vi "Set Channel.vi"(8 "error in (no error)":errorcluster, 10 "ADC Channel Selection":T1, 11 "LINX-ADS1256 in":refnum<class "LINX-ADS1256.lvclass">) -> (0 "error out":errorcluster, 3 "LINX-ADS1256 out":refnum<class "LINX-ADS1256.lvclass">)   [LabVIEW 2020, in "LINX-ADS1256.lvclass"]
uses:
  LINX-ADS1256.lvclass
  Channel Selection.ctl
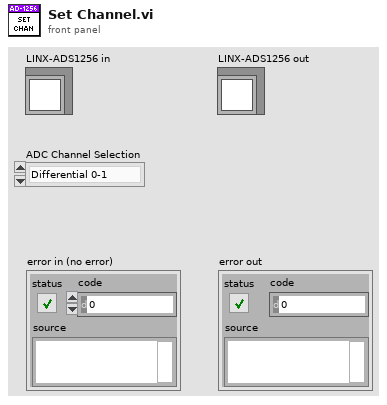
[diagram p1: front panel]
types:
  T1 = typedef "LINX-ADS1256.lvclass/Channel Selection.ctl" = enum16{"Differential 0-1", "Differential 2-3", "Differential 4-5", "Differential 6-7", "Single Ended 0", "Single Ended 1", "Single Ended 2", "Single Ended 3", "Single Ended 4", "Single Ended 5", "Single Ended 6", "Single Ended 7"}
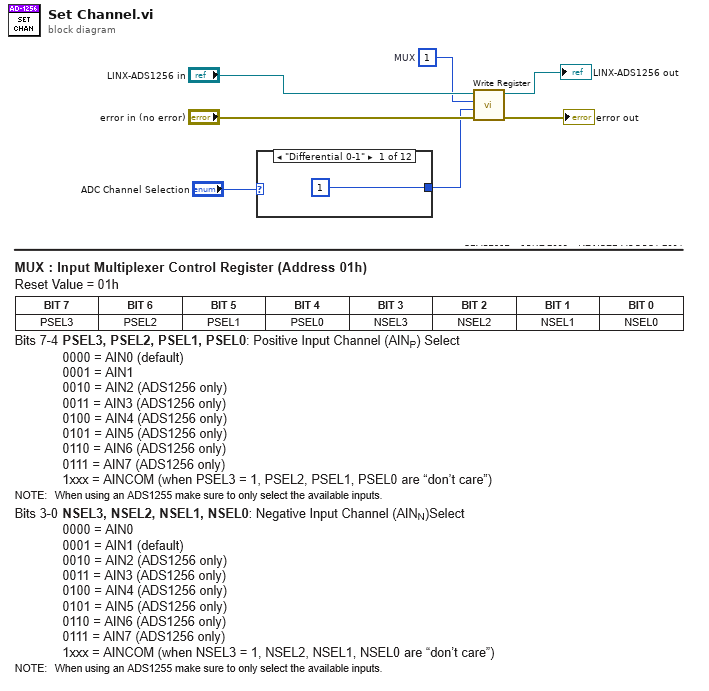
[diagram p0: block diagram]
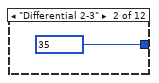
[diagram p2: hidden frame]
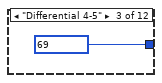
[diagram p3: hidden frame]
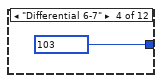
[diagram p4: hidden frame]
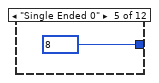
[diagram p5: hidden frame]
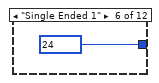
[diagram p6: hidden frame]
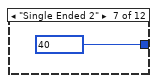
[diagram p7: hidden frame]
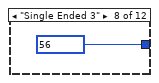
[diagram p8: hidden frame]
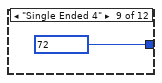
[diagram p9: hidden frame]
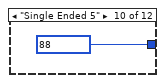
[diagram p10: hidden frame]
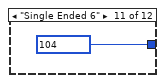
[diagram p11: hidden frame]
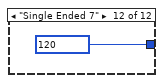
[diagram p12: hidden frame]
diagram:
  w4 = u8 1  # MUX
  n1 = case shown="\"Differential 0-1\"" "ADC Channel Selection" {
    tunnel: [u8 1 ("Data") u8 35 ("Data") u8 69 ("Data") u8 103 ("Data") u8 8 ("Data") u8 24 ("Data") u8 40 ("Data") u8 56 ("Data") u8 72 ("Data") u8 88 ("Data") u8 104 ("Data") u8 120 ("Data")] -> w1
    frame "Differential 0-1" {
    }
    frame "Differential 2-3" {
    }
    frame "Differential 4-5" {
    }
    frame "Differential 6-7" {
    }
    frame "Single Ended 0" {
    }
    frame "Single Ended 1" {
    }
    frame "Single Ended 2" {
    }
    frame "Single Ended 3" {
    }
    frame "Single Ended 4" {
    }
    frame "Single Ended 5" {
    }
    frame "Single Ended 6" {
    }
    frame "Single Ended 7" {
    }
  }
  n2 = call "Write Register.vi"("error in (no error)"="error in (no error)", "Data"=w1, "Register Address"=w4, "LINX-ADS1256 in"="LINX-ADS1256 in") -> ("error out"=→"error out":errorcluster, "LINX-ADS1256 out"=→"LINX-ADS1256 out":refnum<class "LINX-ADS1256.lvclass">)  [unwired: 6 in]
